vi "Write RH_.vi"(8 "error in (no error)":errorcluster, 10 "RH?":bool, 11 "Change Control Value CMD in":refnum<class "Change Control Value CMD.lvclass">) -> (0 "error out":errorcluster, 3 "Change Control Value CMD out":refnum<class "Change Control Value CMD.lvclass">)   [LabVIEW 2014, in "Humidifier Lib.lvlib" / "Change Control Value CMD.lvclass"]
uses:
  Change Control Value CMD.lvclass
  Change Control Value CMD.lvclass/Change Control Value CMD.ctl
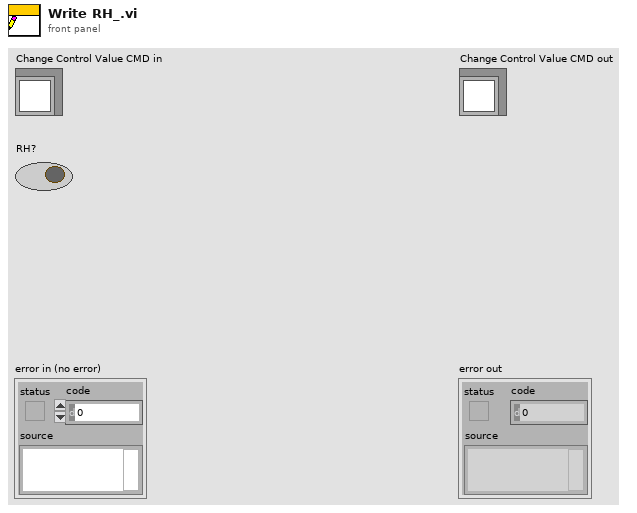
[diagram p1: front panel]
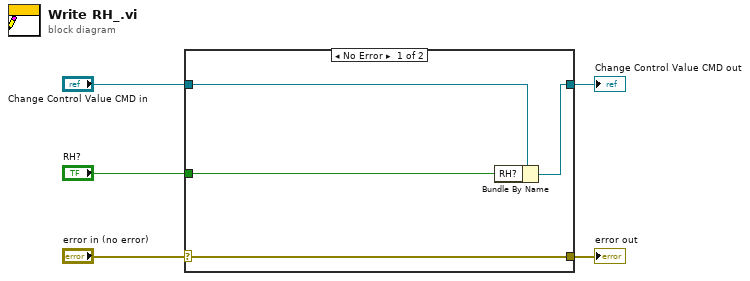
[diagram p0: block diagram]
diagram:
  n1 = case shown="No Error" "error in (no error)" {
    selector: "error in (no error)" -> [w9 w10]
    tunnel: [w9 w10] -> w4
    tunnel: [w7 w11] -> w2
    tunnel: "Change Control Value CMD in" -> [w8 w11]
    tunnel: "RH?" -> [w6 _]
    frame No Error {
      n2 = Bundle By Name(cluster=w8, "RH?"=w6) -> (w7:refnum<class "Change Control Value CMD.lvclass">)
    }
    frame Error {
    }
  }
  "error out" <- w4
  "Change Control Value CMD out" <- w2
